vi "PH_Cont-601k_PowerUnit.Calc State PU.vi"(0 "i ref in":refnum<vi>, 5 "error in (no error)":errorcluster) -> (14 "i ref out":refnum<vi>, 19 "error out":errorcluster)   [LabVIEW 2014, in "PH_Cont-601k_PowerUnit.lvlib"]
doc: "In this VI the state of the PU (running, failure or alarm) is calculated. Depending on the state, several things are done."
uses:
  PH_Cont-601k_PowerUnit.lvlib
  PH_Devices/PH_Cont-601k_PSU/PH_Cont-601k_PSU.Mode.ctl
  PH_Devices/PH_Cont-601k_PSU/PH_Cont-601k_PSU.Readyness Device.ctl
  PH_Basics/PH_StatusHandler/PH_StatusHandler.Status.ctl
  PH_Devices/PH_Cont-601k_PSU/PH_Cont-601k_PSU.lvlib
  PH_Basics/PH_StatusHandler/PH_StatusHandler.lvlib
  PH_Basics/PH_PowerUnit_BaseClass/PH_PowerUnit_BaseClass.lvlib
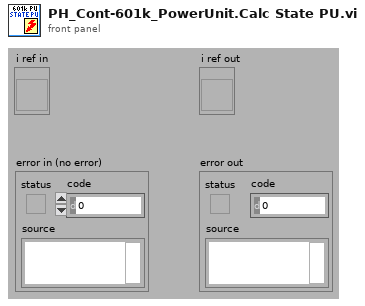
[diagram p1: front panel]
types:
  T1 = typedef "PH_StatusHandler.lvlib/PH_StatusHandler.Status.ctl" = i16
  T2 = typedef "PH_Cont-601k_PSU.lvlib/PH_Cont-601k_PSU.Readyness Device.ctl" = enum32{"OFF", "CONNECTING", "CONNECTED", "OPERATING", "EOC", "ERROR"}
  T3 = enum8{"Enabled", "Disabled", "Disabled and Grayed Out"}
  T4 = typedef "PH_Cont-601k_PSU.lvlib/PH_Cont-601k_PSU.Mode.ctl" = enum32{"STOP", "STANDBY", "READY", "EMISSION", "ERROR"}
  T5 = typedef "PH_Cont-601k_PSU.lvlib/PH_Cont-601k_PSU.i attribute.ctl" = cluster{"GUI Refs":T6, "Interlock":bool, "Service ID applied Voltage":i32, "Device Settings":cluster{"Configuration":T7, "Flash Interval [s]":dbl, "Mode":T4, "Voltage [V]":u16, "Charge":bool, "VISA resource name":refnum<visa-resource-name>}, "Readyness":T8, "Information":cluster{"VISA resource name":refnum<visa-resource-name>, "Tagname Power On":string, "Interlock":cluster{"Instance":string, "Tagname":string}, "Limits [V]":cluster{"Lower":dbl, "Upper":dbl}, "Tagname PSU On":string}, "R2S":bool, "Charge is allowed":bool}
  T6 = typedef "PH_Cont-601k_PSU.lvlib/PH_Cont-601k_PSU.GUI Refs.ctl" = cluster{"Power On":refnum<vi>, "Hard- and Software":refnum<vi>, "Device Status":refnum<vi>, "Device Error":refnum<vi>, "Configuration":refnum<vi>, "Flash Interval [s]":refnum<vi>, "Interlock":refnum<vi>, "Interlock Indicator":refnum<vi>, "Voltage [V]":refnum<vi>, "Readyness":refnum<vi>, "Mode":refnum<vi>, "Reset Error":refnum<vi>, "Expert working":refnum<vi>, "Charge":refnum<vi>, "PSU On":refnum<vi>}
  T7 = typedef "PH_Cont-601k_PSU.lvlib/PH_Cont-601k_PSU.Configuration.ctl" = u16
  T8 = typedef "PH_Cont-601k_PSU.lvlib/PH_Cont-601k_PSU.Readyness.ctl" = cluster{"Program":T9, "Device":T2}
  T9 = typedef "PH_Cont-601k_PSU.lvlib/PH_Cont-601k_PSU.Readyness Program.ctl" = enum32{"OFF", "POWER", "INTERLOCK"}
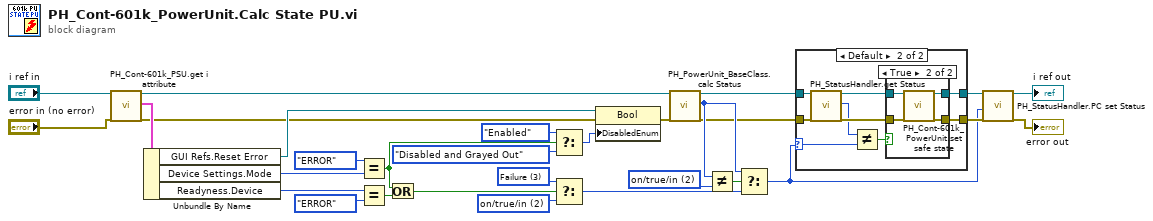
[diagram p0: block diagram]
diagram:
  w1 = T1 2 items=["no info", "off/false/out", "on/true/in", "Failure", "Alarm", "Status 1", "Status 2", "Status 3"] ("Status.Device Status")
  w7 = T1 3 items=["no info", "off/false/out", "on/true/in", "Failure", "Alarm", "Status 1", "Status 2", "Status 3"] ("t")
  w14 = T1 2 items=["no info", "off/false/out", "on/true/in", "Failure", "Alarm", "Status 1", "Status 2", "Status 3"] ("y")
  n1 = call "PH_Cont-601k_PSU.get i attribute.vi"("i ref in"="i ref in", "error in (no error)"="error in (no error)") -> ("i ref out"=w6:refnum<vi>, "i attribute"=w18:T5, "error out"=w17:errorcluster)  [unwired: 15 in]
  n2 = Unbundle By Name(w18) -> ("GUI Refs.Reset Error"=w21:refnum<vi>, "Device Settings.Mode"=w19:T4, "Readyness.Device"=w26:T2)
  n3 = Equal?(x=PH_Cont-601k_PSU.Mode."ERROR" ("Device Setings.Mode"), y=w19) -> (x = y?=w11:bool)
  n4 = Equal?(x=w26, y=PH_Cont-601k_PSU.Readyness_Device."ERROR" ("Readyness.Device")) -> (x = y?=w10:bool)
  n5 = Or(x=w11, y=w10) -> (x .or. y?=w9:bool)
  n6 = Select(t=T3."Enabled" ("Disabled"), s=w11, f=T3."Disabled and Grayed Out") -> (s? t:f=w23:T3)
  n7 = Select(t=w7, s=w9, f=w1) -> (s? t:f=w8:T1)
  n8 = property class="Bool"(reference=w21, error in=w17, "DisabledEnum"=w23) -> (error out=w5:errorcluster)  [unwired: 1 out]
  n9 = call "PH_PowerUnit_BaseClass.calc Status.vi"("VI in"=w6, "error in (no error)"=w5) -> ("VI out"=w4:refnum<vi>, "PU Status"=w12:T1, "error out"=w3:errorcluster)  [unwired: 15 in]
  n10 = Not Equal?(x=w12, y=w14) -> (x != y?=w13:bool)
  n11 = Select(t=w12, s=w13, f=w8) -> (s? t:f=w2:T1)
  n12 = case shown="Default" w2 {
    selector: w2 -> [_ w34]
    tunnel: [w32 w41] -> w16
    tunnel: [w31 w40] -> w15
    tunnel: w4 -> [w32 w39]
    tunnel: w3 -> [w31 w37]
    frame 2 {
    }
    frame Default {
      n13 = call "PH_StatusHandler.get Status.vi"("VI in"=w39, "error in"=w37) -> ("VI out"=w38:refnum<vi>, "Status"=w33:T1, "error out"=w36:errorcluster)  [unwired: 15 in]
      n14 = Not Equal?(x=w33, y=w34) -> (x != y?=w35:bool)
      n15 = case shown="True" w35 {
        tunnel: w38 -> [w43 w47]
        tunnel: w36 -> [w42 w46]
        tunnel: [w43 w45] -> w41
        tunnel: [w42 w44] -> w40
        frame False {
        }
        frame True {
          n16 = call "PH_Cont-601k_PowerUnit.set safe state.vi"("i ref in"=w47, "error in (no error)"=w46) -> ("i ref out"=w45:refnum<vi>, "error out"=w44:errorcluster)  [unwired: 16 in]
        }
      }
    }
  }
  n17 = call "PH_StatusHandler.PC set Status.vi"("i ref in"=w16, "Status"=w2, "error in (no error)"=w15) -> ("i ref out"=→"i ref out":refnum<vi>, "error out"=→"error out":errorcluster)  [unwired: 15 in]
